vi "Connect.vi"(8 "error in (no error)":errorcluster, 10 "Channel(s)":string, 11 "Sim Switch in":refnum<class "Sim Switch.lvclass">) -> (0 "error out":errorcluster, 3 "Sim Switch out":refnum<class "Sim Switch.lvclass">)   [LabVIEW 2019, in "Concrete.lvlib" / "Sim Switch.lvclass"]
uses:
  Sim Switch.lvclass
  Harware Abstraction/Switch/Switch.lvclass
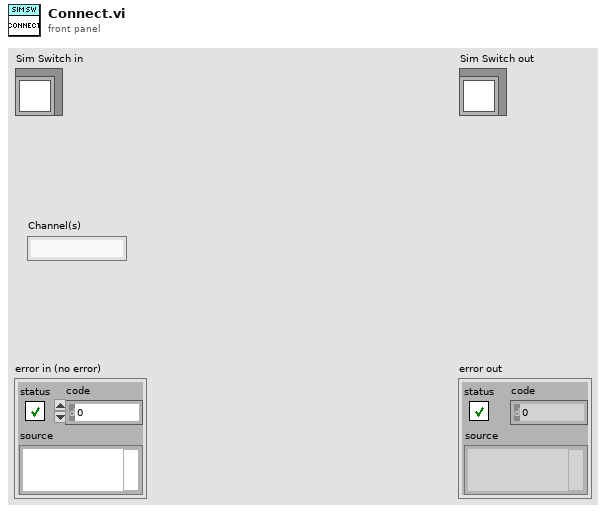
[diagram p1: front panel]
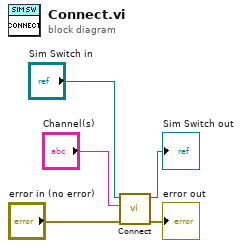
[diagram p0: block diagram]
diagram:
  n1 = call-parent "Connect.vi"("error in (no error)"="error in (no error)", "Channel(s)"="Channel(s)", "Switch in"="Sim Switch in") -> ("error out"=→"error out":errorcluster, "Switch out"=→"Sim Switch out":refnum<class "Sim Switch.lvclass">)  [unwired: 7 in]
